vi "FRCts20_Backend_EventRoot_POST.vi"(6 "Message Attributes":T4, 8 "error in (no error)":errorcluster, 10 "Data":string, 11 "Engine_Refnums":T1) -> (0 "error out":errorcluster)   [LabVIEW 2013, in "FRCts20_Backend_Engine.lvlib"]
doc: "Adds a new event, called by the Event Root API. Expects an event name, start time, and end time."
uses:
  FRCts20_Backend_Engine.lvlib
  Dependencies/Keyed Array/KeyedArray.ctl
  FRCts20_Backend_EngineRefnums.ctl
  INI_Accessor/FRCts20_Backend_INI Controller.lvclass
  Dependencies/AMC/_SubVIs/TypeDefs/Message Queue.ctl
  Dependencies/AMC/_SubVIs/TypeDefs/Message.ctl
  <vilib>/addons/database/Connection.llb/Conn ObjectReference.ctl
  FRCts20_Backend_FGVOperation.ctl
  FRCts20_Backend_API/FRCts20_Backend_API_EventRoot.ctl
  FRCts20_Backend_API/FRCts20_Backend_API.lvlib
  Dependencies/Keyed Array/Tools_KeyedArray.lvlib
  Dependencies/AMC/AMC.lvlib
  <vilib>/addons/database/NI_Database_API.lvlib
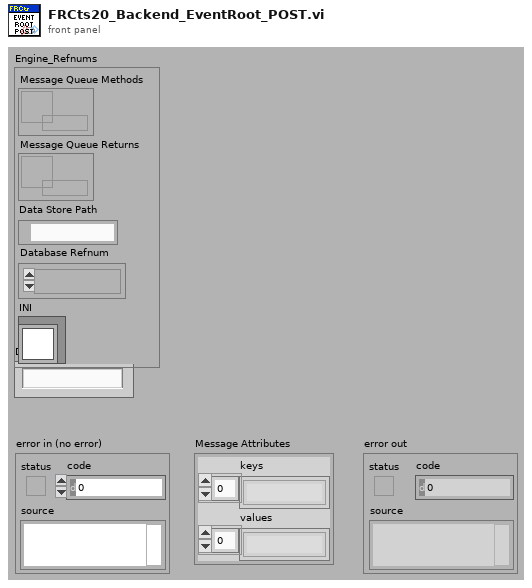
[diagram p1: front panel]
types:
  T1 = typedef "FRCts20_Backend_Engine.lvlib/FRCts20_Backend_EngineRefnums.ctl" = cluster{"Message Queue Methods":T2, "Message Queue Returns":T2, "Data Store Path":path, "Database Refnum":T3, "INI":refnum<class "FRCts20_Backend_INI Controller.lvclass">}
  T2 = typedef "AMC.lvlib/Message Queue.ctl" = refnum<queue>
  T3 = typedef "NI_Database_API.lvlib/Conn ObjectReference.ctl" = refnum<k1>
  T4 = typedef "Tools_KeyedArray.lvlib/KeyedArray.ctl" = cluster{"keys":string[], "values":string[]}
  T5 = typedef "FRCts20_Backend_API.lvlib/FRCts20_Backend_API_EventRoot.ctl" = cluster{"Event":cluster{"Event Index":u32, "Event Name":string, "Start Time":timestamp, "End Time":timestamp, "OpenIssues":u8, "IsLive":bool}[], "APIReturn":string}
  T6 = typedef "FRCts20_Backend_Engine.lvlib/FRCts20_Backend_FGVOperation.ctl" = enum16{"Initialize", "EnqueueMessage", "EnqueueDataReturn", "FlushMessage", "FlushDataReturn"}
  T7 = cluster{"Event Index":u32, "Event Name":string, "Start Time":timestamp, "End Time":timestamp, "OpenIssues":u8, "IsLive":bool}[]
  T8 = cluster{"Event Index":u32, "Event Name":string, "Start Time":timestamp, "End Time":timestamp, "OpenIssues":u8, "IsLive":bool}
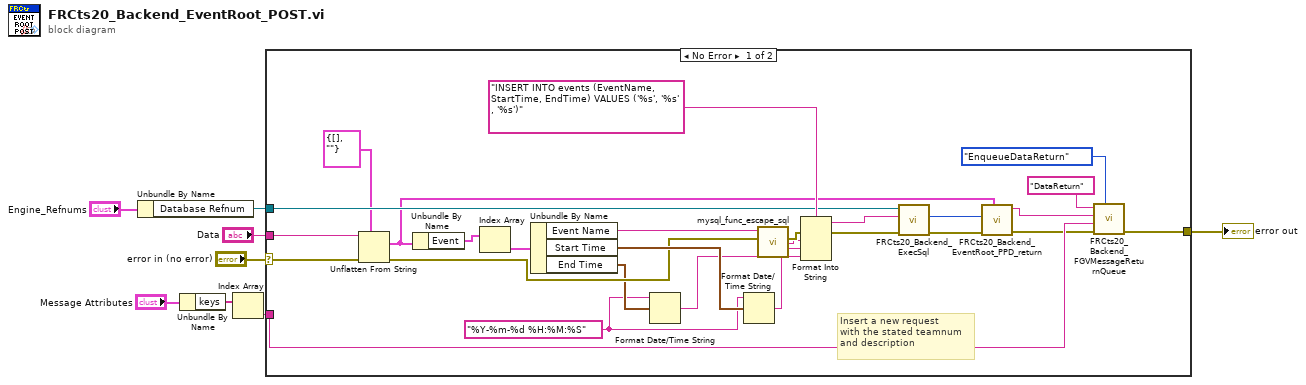
[diagram p0: block diagram]
diagram:
  n1 = Unbundle By Name("Engine_Refnums") -> ("Database Refnum"=w5:T3)
  n2 = Unbundle By Name("Message Attributes") -> ("keys"=w2:string[])
  n3 = Index Array(array=w2) -> (element=w1:string)  [unwired: 1 in]
  n4 = case shown="No Error" "error in (no error)" {
    selector: "error in (no error)" -> [w32 w36]
    tunnel: [w35 w36] -> w7
    tunnel: w5 -> [w23 _]
    tunnel: "Data" -> [w33 _]
    tunnel: w1 -> [w34 _]
    frame No Error {
      w9 = "%Y-%m-%d %H:%M:%S" ("time format string (%c)")
      # "Insert a new request\nwith the stated teamnum\nand description"
      n5 = Unflatten From String(type=T5 {"Event"=[], "APIReturn"=""} ("Competition"), binary string=w33, error in (no error)=w32) -> (value=w10:T5, error out=w27:errorcluster)  [unwired: 2 in, 1 out]
      n6 = Unbundle By Name(w10) -> ("Event"=w12:T7)
      n7 = Index Array(array=w12) -> (element=w11:T8)  [unwired: 1 in]
      n8 = Unbundle By Name(w11) -> ("Event Name"=w26:string, "Start Time"=w28:timestamp, "End Time"=w15:timestamp)
      n9 = Format Date/Time String(time format string (%c)=w9, seconds (now)=w15) -> (date/time string=w14:string)  [unwired: 1 in]
      n10 = Format Date/Time String(time format string (%c)=w9, seconds (now)=w28) -> (date/time string=w16:string)  [unwired: 1 in]
      n11 = call "mysql_func_escape_sql.vi"("error in (no error)"=w27, "sqlin"=w26) -> ("error out"=w25:errorcluster, "escaped"=w24:string)  [unwired: 8 in]
      n12 = Format Into String(format string="INSERT INTO events (EventName, StartTime, EndTime) VALUES ('%s', '%s' , '%s')", error in=w25, w24, w16, w14) -> (resulting string=w22:string, error out=w21:errorcluster)  [unwired: 1 in]
      n13 = call "FRCts20_Backend_ExecSql.vi"("error in (no error)"=w21, "format string"=w22, "Refnum in"=w23) -> ("error out"=w19:errorcluster, "rows affected"=w20:i32)  [unwired: 6 in, 1 out]
      n14 = call "FRCts20_Backend_EventRoot_PPD_return.vi"("Events"=w10, "error in (no error)"=w19, "rows affected"=w20) -> ("error out"=w18:errorcluster, "data string"=w17:string)  [unwired: 7 in]
      n15 = call "FRCts20_Backend_FGVMessageReturnQueue.vi"("Operation"=FRCts20_Backend_FGVOperation."EnqueueDataReturn", "error in (no error)"=w18, "Key"=w34, "Message Value"=w17, "Message Name"="DataReturn") -> ("error out"=w35:errorcluster)  [unwired: 5 in, 1 out]
    }
    frame Error {
    }
  }
  "error out" <- w7
